vi "Write Customer Name.vi"(10 "Customer Name":string, 11 "Condiment Decorator in":refnum<class "Condiment Decorator.lvclass">) -> (3 "Condiment Decorator in 2":refnum<class "Condiment Decorator.lvclass">)   [LabVIEW 2013, in "Condiment Decorator.lvclass"]
uses:
  Condiment Decorator.lvclass
  Condiment Decorator.lvclass/Condiment Decorator.ctl
  Abstract Beverage/Abstract Beverage.lvclass
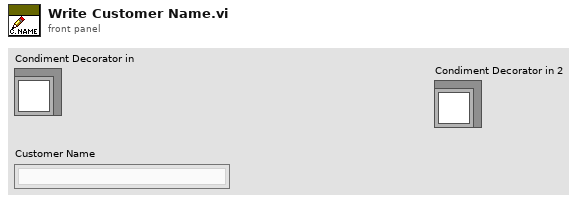
[diagram p1: front panel]
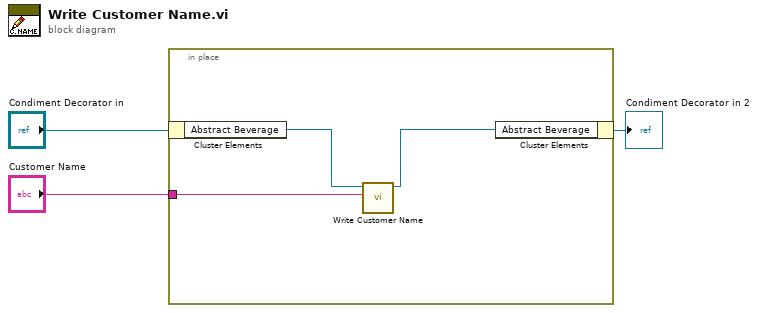
[diagram p0: block diagram]
diagram:
  n1 = in-place {
    in-place-border: "Customer Name" -> [w4]
    n2 = in-place-cluster #1("Condiment Decorator in") -> ("Abstract Beverage"=w6:refnum<class "Abstract Beverage.lvclass">)
    n3 = call-dynamic "Write Customer Name.vi"("Customer Name"=w4, "Abstract Beverage in"=w6) -> ("Abstract Beverage in 2"=w5:refnum<class "Abstract Beverage.lvclass">)  [unwired: 9 in]
    n4 = in-place-cluster #1("Abstract Beverage"=w5) -> (→"Condiment Decorator in 2":refnum<class "Condiment Decorator.lvclass">)
  }
